vi "Teleop.vi"(10 "Match Info":T1={"Autonomous Elapsed Seconds"=0.0, "TeleOp Elapsed Seconds"=0.0, "Disabled Elapsed Seconds"=0.0, "Visited Autonomous"=FALSE, "Visited TeleOp"=FALSE, "Visited Disabled"=FALSE, "Autonomous Settings"={"Autonomous Style"=enum."Independent", "VI Refnum"=refnum}}, 11 "Call Context":T2) -> ()   [LabVIEW 2015]
doc: "This VI is called for each TeleOp packet received from the DS where the robot is not disabled. It is often used to read from the joysticks and update I/O or to update setpoints for timed control loops. It should complete and return within 20 milliseconds or it may miss DS packets."
uses:
  <vilib>/Rock Robotics/WPI/DriverStation/WPI_DriverStationDerivedRobotMode.ctl
  <vilib>/Rock Robotics/WPI/DriverStation/WPI_DriverStationMatch Info.ctl
  <vilib>/Rock Robotics/WPI/Solenoid/WPI_SolenoidValue.ctl
  <vilib>/Rock Robotics/WPI/CAN/TalonSRX/WPI_CANTalonSRX_BrakeOverride.ctl
  <vilib>/Rock Robotics/WPI/Utilities/WPI_GetSetVariantRefNum.vi
  <vilib>/Rock Robotics/Network Tables/NT Write Boolean Array.vi
  <vilib>/Rock Robotics/Network Tables/NT Write Numeric Array.vi
  <vilib>/Rock Robotics/WPI/Solenoid/WPI_SolenoidSetEnum.vi
  <vilib>/Rock Robotics/Network Tables/NT Read Boolean.vi
  <vilib>/addons/control/pid/pid.llb/PID (DBL).vi
  ADI MXP IMU/ADI MXP IMU/FRC ADI MXP IMU.lvlib
  <vilib>/addons/control/pid/NI_PID_pid.lvlib
panel:
  out "IMU AHRS":cluster{"Pitch":dbl, "Roll":dbl, "Yaw":dbl}
  out "IMU AHRS DELTA":cluster{"Pitch":dbl, "Roll":dbl, "Yaw":dbl}
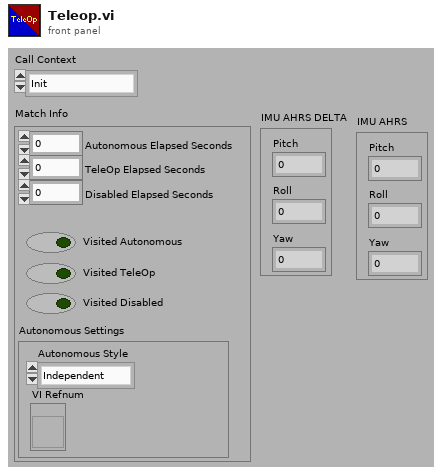
[diagram p1: front panel]
types:
  T1 = typedef "WPI_DriverStationMatch Info.ctl" = cluster{"Autonomous Elapsed Seconds":dbl, "TeleOp Elapsed Seconds":dbl, "Disabled Elapsed Seconds":dbl, "Visited Autonomous":bool, "Visited TeleOp":bool, "Visited Disabled":bool, "Autonomous Settings":cluster{"Autonomous Style":enum16{"Iterative", "Independent"}, "VI Refnum":refnum<vi>}}
  T2 = typedef "WPI_DriverStationDerivedRobotMode.ctl" = enum16{"Init", "Execute", "Stop"}
  T3 = typedef "WPI_CANTalonSRX_BrakeOverride.ctl" = enum8{"No Override", "Override to Coast", "Override to Brake"}
  T4 = typedef "WPI_SolenoidValue.ctl" = enum16{"Off", "On", "Forward", "Reverse"}
  T5 = typedef "WPI_MotorControlDeviceRef.ctl" = cluster{"DeviceStatus":errorcluster, "Type":T6, "PWM":cluster{"PWM Channel":T7, "DeadBand":T8}, "CAN":cluster{"Device Number":u8, "Control Mode":T9, "Semaphore":T10, "Max Vout":dbl, "TalonSRX Control Mode":T11}, "Invert":bool}
  T6 = typedef "WPI_MotorControlType.ctl" = enum16{"PWM", "CAN", "CANTalonSRX"}
  T7 = typedef "FPGA_DIOPWMChannel.ctl" = enum8{"PWM 0", "PWM 1", "PWM 2", "PWM 3", "PWM 4", "PWM 5", "PWM 6", "PWM 7", "PWM 8", "PWM 9", "PWM MXP 0", "PWM MXP 1", "PWM MXP 2", "PWM MXP 3", "PWM MXP 4", "PWM MXP 5", "PWM MXP 6", "PWM MXP 7", "PWM MXP 8", "PWM MXP 9", "Invalid"}
  T8 = typedef "WPI_PWMDeadband.ctl" = cluster{"Name":string, "maxPositivePwm":i32, "minPositivePwm":i32, "centerPwm":i32, "maxNegativePwm":i32, "minNegativePwm":i32, "angularRange":u16}
  T9 = typedef "WPI_CANJaguar_ControlMode.ctl" = enum8{"Percent VBus", "Current", "Speed", "Position", "Voltage"}
  T10 = typedef "Semaphore RefNum" = refnum<k1>
  T11 = typedef "WPI_CANTalonSRX_APIControlMode.ctl" = enum8{"Percent VBus", "Speed", "Position", "Slave", "Unchanged / Invalid", "Voltage Compensation", "Current", "Motion Profile"}
  T12 = typedef "FRC ADI MXP IMU.lvlib/WPI_AnalogDevicesIMUInterruptDevRef.ctl" = cluster{"SimpleGyroDevRef":T13, "InterruptRef":T15}
  T13 = typedef "FRC ADI MXP IMU.lvlib/WPI_AnalogDevicesIMUDevRef.ctl" = cluster{"DevStatus":errorcluster, "Handle":i32, "SPI Bus":T14, "Device Found":bool, "Sample Rate":dbl, "Device Ready":bool, "Yaw Axis":enum16{"X", "Y", "Z"}, "AHRS Algorithm":enum16{"Complementary", "Madgwick"}}
  T14 = typedef "spi_bus.ctl" = enum16{"SPI On-Board, CS0", "SPI On-Board, CS1", "SPI On-Board, CS2", "SPI On-Board, CS3", "SPI MXP", "Invalid"}
  T15 = typedef "WPI_InterruptRef.ctl" = cluster{"DevStatus":errorcluster, "InterruptIndex":T16}
  T16 = typedef "FPGA_InterruptIndex.ctl" = enum8{"0", "1", "2", "3", "4", "5", "6", "7", "Invalid"}
  T17 = typedef "WPI_JoystickDevRef.ctl" = cluster{"Device":T18}
  T18 = typedef "WPI_JoystickDeviceEnum.ctl" = enum16{"USB 0", "USB 1", "USB 2", "USB 3", "USB 4", "USB 5"}
  T19 = cluster{"proportional gain (Kc)":dbl, "integral time (Ti, min)":dbl, "derivative time (Td, min)":dbl}
  T20 = typedef "WPI_SwitchDevRef.ctl" = cluster{"DevStatus":errorcluster, "DIO Channel":T21, "CntIndex":T22, "Normally Closed":bool}
  T21 = typedef "FPGA_DIOChannel.ctl" = enum8{"DIO 0", "DIO 1", "DIO 2", "DIO 3", "DIO 4", "DIO 5", "DIO 6", "DIO 7", "DIO 8", "DIO 9", "DIO MXP 0", "DIO MXP 1", "DIO MXP 2", "DIO MXP 3", "DIO MXP 4", "DIO MXP 5", "DIO MXP 6", "DIO MXP 7", "DIO MXP 8", "DIO MXP 9", "DIO MXP 10", "DIO MXP 11", "DIO MXP 12", "DIO MXP 13", "DIO MXP 14", "DIO MXP 15", "Invalid"}
  T22 = typedef "FPGA_CounterCtrSystemIndex.ctl" = enum8{"Ctr 0", "Ctr 1", "Ctr 2", "Ctr 3", "Ctr 4", "Ctr 5", "Ctr 6", "Ctr 7", "Invalid"}
  T23 = typedef "WPI_SolenoidDevRef.ctl" = cluster{"DevStatus":errorcluster, "Pneumatics Control Module":u8, "Forward Solenoid Channel":T24, "Reverse Solenoid Channel":T24}
  T24 = typedef "WPI_SolenoidChannel.ctl" = enum8{"Solenoid 0", "Solenoid 1", "Solenoid 2", "Solenoid 3", "Solenoid 4", "Solenoid 5", "Solenoid 6", "Solenoid 7", "Invalid"}
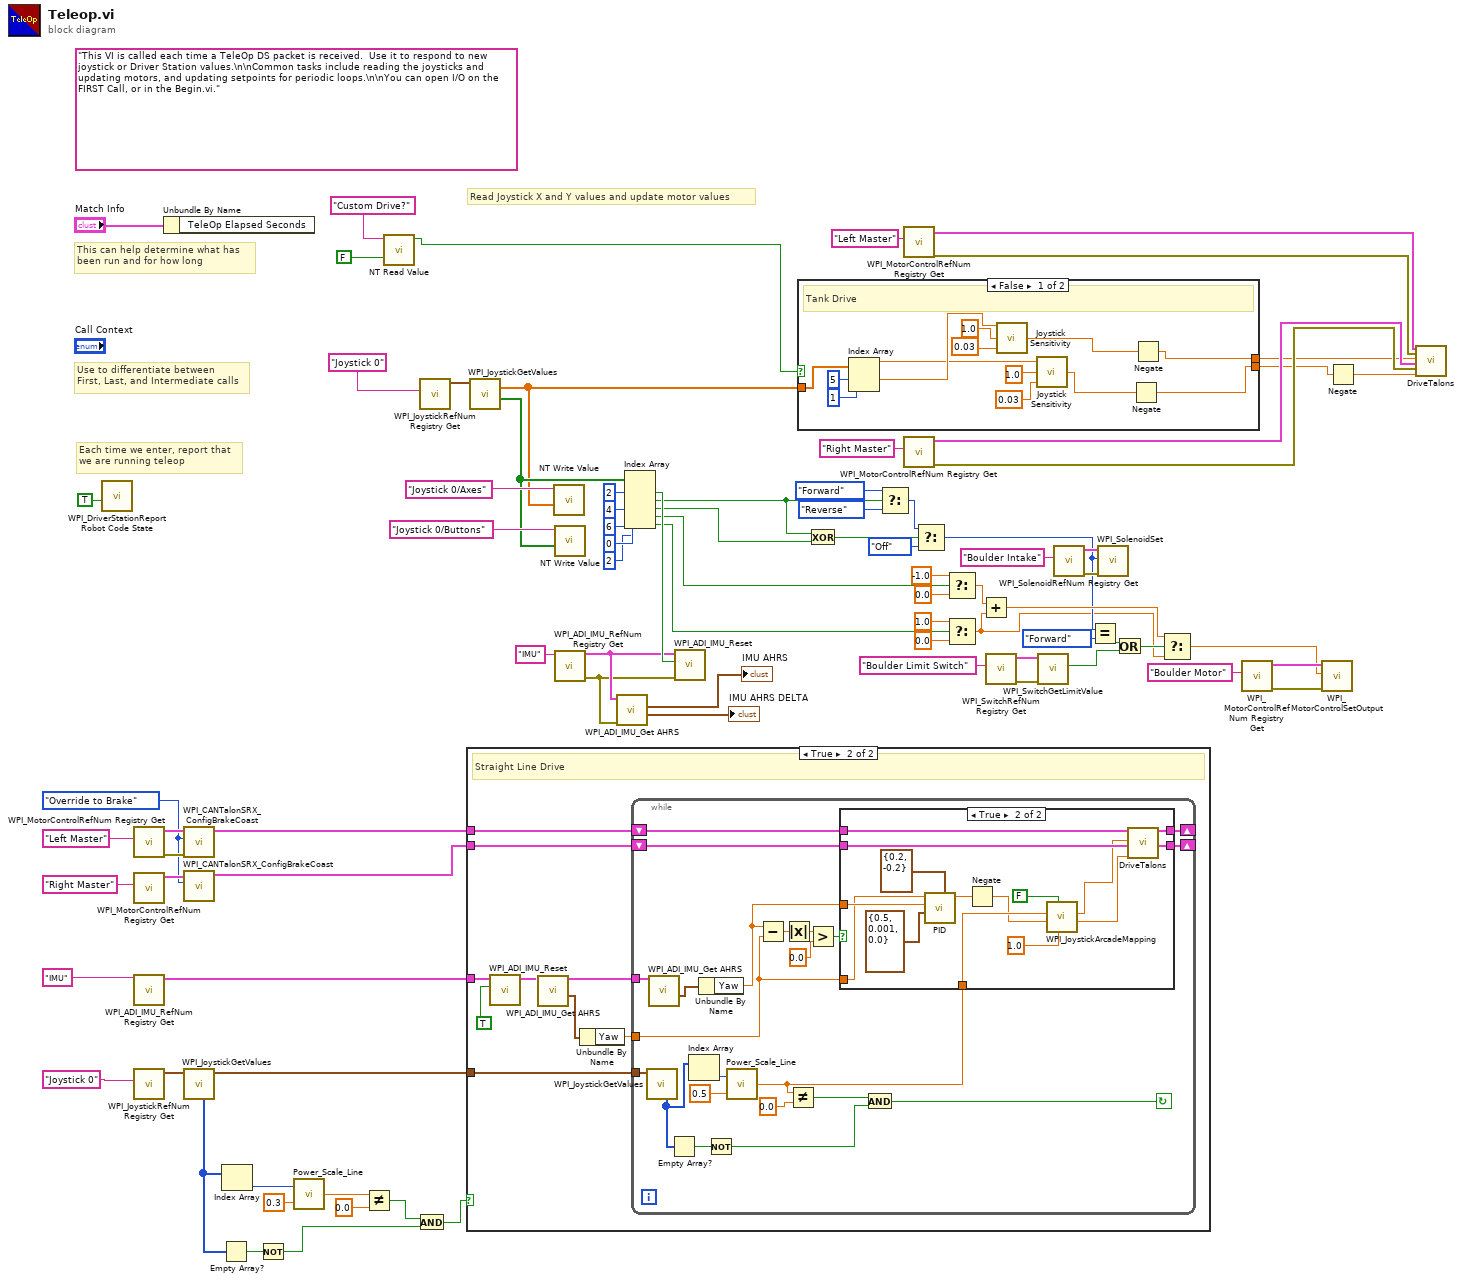
[diagram p0: block diagram]
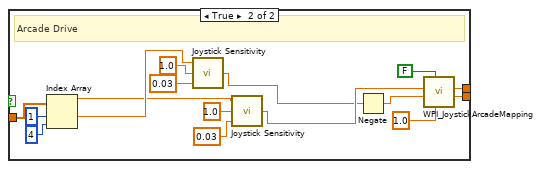
[diagram p2: hidden frame]
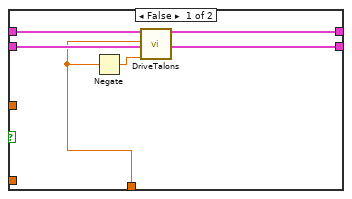
[diagram p4: hidden frame]
diagram:
  w34 = WPI_CANTalonSRX_BrakeOverride."Override to Brake" ("Brake / Coast Mode")
  (unwired) "This VI is called each time a TeleOp DS packet is received.  Use it to respond to new joystick or Driver Station values.\n\nCommon tasks include reading the joysticks and updating motors, and updating setpoints for periodic loops.\n\nYou can open I/O on the FIRST Call, or in the Begin.vi."
  # "Each time we enter, report that\nwe are running teleop"
  # "Use to differentiate between\nFirst, Last, and Intermediate calls"
  # "This can help determine what has\nbeen run and for how long"
  # "Read Joystick X and Y values and update motor values"
  n1 = call <vilib>:"WPI_DriverStationReport Robot Code State.vi"("TeleOp"=TRUE ("Autonomous")) -> ()  [unwired: 10 in, 1 out]
  n2 = call <vilib>:"WPI_MotorControlRefNum Registry Get.vi"("refnum name"="Left Master") -> ("error out"=w36:errorcluster, "MotorControlDevRef"=w37:T5)  [unwired: 9 in]
  n3 = call <vilib>:"WPI_MotorControlRefNum Registry Get.vi"("refnum name"="Right Master") -> ("MotorControlDevRef"=w35:T5)  [unwired: 9 in, 1 out]
  n4 = call "WPI_ADI_IMU_RefNum Registry Get.vi"("refnum name"="IMU") -> ("ADI IMU Interrupt DevRef"=w18:T12)  [unwired: 9 in, 1 out]
  n5 = call <vilib>:"WPI_JoystickRefNum Registry Get.vi"("refnum name"="Joystick 0") -> ("JoystickDevRef"=w13:T17)  [unwired: 1 in, 9 out]
  n6 = Unbundle By Name("Match Info") -> ()  [unwired: 1 out]
  n7 = call <vilib>:"WPI_CANTalonSRX_ConfigBrakeCoast.vi"("error in (no error)"=w36, "Brake / Coast Mode"=w34, "CAN Talon SRX Ref"=w37) -> ("CAN Talon SRX Ref"=w16:T5)  [unwired: 7 in, 1 out]
  n8 = call <vilib>:"WPI_CANTalonSRX_ConfigBrakeCoast.vi"("Brake / Coast Mode"=w34, "CAN Talon SRX Ref"=w35) -> ("CAN Talon SRX Ref"=w17:T5)  [unwired: 8 in, 1 out]
  n9 = call <vilib>:"WPI_JoystickGetValues.vi"("JoystickDevRef"=w13) -> ("JoystickDevRef"=w12:T17, "POVs"=w7:i16[])  [unwired: 6 in, 3 out]
  n10 = Empty Array?(array=w7) -> (empty?=w6:bool)
  n11 = Index Array(array=w7) -> (element=w15:i16)  [unwired: 1 in]
  n12 = Not(x=w6) -> (.not. x?=w5:bool)
  n13 = call "Power_Scale_Line.vi"("Power Input"=0.3, "POV"=w15) -> ("Power Output"=w19:dbl)
  n14 = Not Equal?(x=w19, y=0.0) -> (x != y?=w4:bool)
  n15 = call-poly <vilib>:"NT Read Value.vi"("Default Value"=FALSE, "Name"="Custom Drive?") -> ("Boolean"=w21:bool)  [unwired: 8 in, 1 out]
  n16 = And(x=w4, y=w5) -> (x .and. y?=w3:bool)
  n17 = call <vilib>:"WPI_JoystickRefNum Registry Get.vi"("refnum name"="Joystick 0") -> ("JoystickDevRef"=w31:T17)  [unwired: 1 in, 9 out]
  n18 = case shown="True" w3 {
    tunnel: w18 -> [_ w87]
    tunnel: w17 -> [_ w92]
    tunnel: w16 -> [_ w91]
    tunnel: w12 -> [_ w90]
    frame False {
      # "POV Not Pressed"
    }
    frame True {
      # "Straight Line Drive"
      n19 = call "WPI_ADI_IMU_Reset.vi"("Reset? (T)"=TRUE, "ADI IMU Interrupt DevRef"=w87) -> ("ADI IMU Interrupt DevRef Out"=w86:T12)  [unwired: 8 in, 1 out]
      n20 = call "WPI_ADI_IMU_Get AHRS.vi"("ADI IMU Interrupt DevRef"=w86) -> ("IMU AHRS DELTA"=w88:cluster{"Pitch":dbl, "Roll":dbl, "Yaw":dbl}, "ADI IMU Interrupt DevRef Out"=w89:T12)  [unwired: 6 in, 3 out]
      n21 = Unbundle By Name(w88) -> ("Yaw"=w93:dbl)
      n22 = while {
        tunnel: w89 -> [w97]
        tunnel: w93 -> [w106]
        shift-right: [w111] -> _
        shift-left: w92 -> [w110]
        shift-right: [w112] -> _
        shift-left: w91 -> [w109]
        tunnel: w90 -> [w103]
        stop <- w99 continue-if-true
        n23 = call <vilib>:"WPI_JoystickGetValues.vi"("JoystickDevRef"=w103) -> ("POVs"=w98:i16[])  [unwired: 6 in, 4 out]
        n24 = call "WPI_ADI_IMU_Get AHRS.vi"("ADI IMU Interrupt DevRef"=w97) -> ("IMU AHRS DELTA"=w96:cluster{"Pitch":dbl, "Roll":dbl, "Yaw":dbl})  [unwired: 6 in, 4 out]
        n25 = Empty Array?(array=w98) -> (empty?=w102:bool)
        n26 = Index Array(array=w98) -> (element=w113:i16)  [unwired: 1 in]
        n27 = Unbundle By Name(w96) -> ("Yaw"=w107:dbl)
        n28 = Not(x=w102) -> (.not. x?=w101:bool)
        n29 = call "Power_Scale_Line.vi"("Power Input"=0.5, "POV"=w113) -> ("Power Output"=w108:dbl)
        n30 = Subtract(x=w107, y=w106) -> (x-y=w95:dbl)
        n31 = Absolute Value(x=w95) -> (abs(x)=w94:dbl)
        n32 = Not Equal?(x=w108, y=0.0) -> (x != y?=w100:bool)
        n33 = Greater?(x=w94, y=0.0) -> (0:w104:bool)
        n34 = case shown="True" w104 {
          tunnel: [w121 w136] -> w112
          tunnel: [w120 w135] -> w111
          tunnel: w110 -> [w118 w134]
          tunnel: w109 -> [w119 w133]
          tunnel: w108 -> [w116 w125]
          tunnel: w107 -> [_ w132]
          tunnel: w106 -> [_ w131]
          frame False {
            n35 = Negate(x=w116) -> (-x=w117:dbl)
            n36 = call "DriveTalons.vi"("Left Motor"=w119, "Left Stick"=w116, "Right Motor"=w118, "Right Stick"=w117) -> ("Left Motor Out"=w121:T5, "Right Motor Out"=w120:T5)  [unwired: 12 in, 2 out]
          }
          frame True {
            n37 = call-poly <vilib>:"PID.vi"("output range"=cluster{"output high":dbl, "output low":dbl} {"output high"=0.2, "output low"=-0.2}, "PID gains"=T19 {"proportional gain (Kc)"=0.5, "integral time (Ti, min)"=0.001, "derivative time (Td, min)"=0.0}, "process variable"=w132, "setpoint"=w131) -> ("output"=w124:dbl)  [unwired: 6 in, 1 out]
            n38 = Negate(x=w124) -> (-x=w123:dbl)
            n39 = call <vilib>:"WPI_JoystickArcadeMapping.vi"("Max Output"=1.0, "Square Inputs"=FALSE, "Y axis value"=w123, "X axis value"=w125) -> ("Right Motor Value"=w126:dbl, "Left Motor Value"=w122:dbl)  [unwired: 6 in]
            n40 = call "DriveTalons.vi"("Left Motor"=w133, "Left Stick"=w122, "Right Motor"=w134, "Right Stick"=w126) -> ("Left Motor Out"=w136:T5, "Right Motor Out"=w135:T5)  [unwired: 12 in, 2 out]
          }
        }
        n41 = And(x=w100, y=w101) -> (x .and. y?=w99:bool)
      }
    }
  }
  n42 = call <vilib>:"WPI_JoystickGetValues.vi"("JoystickDevRef"=w31) -> ("Buttons"=w78:bool[], "Axes"=w20:dbl[])  [unwired: 6 in, 3 out]
  n43 = call-poly <vilib>:"NT Write Value.vi"("Numeric Array"=w20, "Name"="Joystick 0/Axes") -> ()  [unwired: 9 in, 1 out]
  n44 = call-poly <vilib>:"NT Write Value.vi"("Boolean Array"=w78, "Name"="Joystick 0/Buttons") -> ()  [unwired: 9 in, 1 out]
  n45 = call "WPI_ADI_IMU_RefNum Registry Get.vi"("refnum name"="IMU") -> ("error out"=w10:errorcluster, "ADI IMU Interrupt DevRef"=w11:T12)  [unwired: 9 in]
  n46 = call "WPI_ADI_IMU_Get AHRS.vi"("error in"=w10, "ADI IMU Interrupt DevRef"=w11) -> ("IMU AHRS DELTA"=→"IMU AHRS DELTA":cluster{"Pitch":dbl, "Roll":dbl, "Yaw":dbl}, "IMU AHRS"=→"IMU AHRS":cluster{"Pitch":dbl, "Roll":dbl, "Yaw":dbl})  [unwired: 5 in, 3 out]
  n47 = Index Array(array=w78, index #1=2 ("index"), index #2=4 ("index"), index #3=6 ("index"), index #4=0 ("index"), index #5=2 ("index")) -> (element #1=w76:bool, element #2=w41:bool, element #3=w42:bool, element #4=w53:bool, element #5=w52:bool)
  n48 = call "WPI_ADI_IMU_Reset.vi"("error in"=w10, "Reset? (T)"=w76, "ADI IMU Interrupt DevRef"=w11) -> ()  [unwired: 7 in, 2 out]
  n49 = case shown="False" w21 {
    tunnel: [w139 w163] -> w22
    tunnel: [w137 w162] -> w2
    tunnel: w20 -> [w147 w159]
    frame False {
      # "Tank Drive"
      n50 = Index Array(array=w147, index #1=5 ("index"), index #2=1 ("index")) -> (element #1=w146:dbl, element #2=w143:dbl)
      n51 = call "Joystick Sensitivity.vi"("B"=0.03, "A"=1.0, "X"=w146) -> ("Y"=w140:dbl)
      n52 = call "Joystick Sensitivity.vi"("B"=0.03, "A"=1.0, "X"=w143) -> ("Y"=w138:dbl)
      n53 = Negate(x=w138) -> (-x=w137:dbl)
      n54 = Negate(x=w140) -> (-x=w139:dbl)
    }
    frame True {
      # "Arcade Drive"
      n55 = Index Array(array=w159, index #1=1 ("index"), index #2=4 ("index")) -> (element #1=w158:dbl, element #2=w155:dbl)
      n56 = call "Joystick Sensitivity.vi"("B"=0.03, "A"=1.0, "X"=w158) -> ("Y"=w151:dbl)
      n57 = call "Joystick Sensitivity.vi"("B"=0.03, "A"=1.0, "X"=w155) -> ("Y"=w152:dbl)
      n58 = Negate(x=w151) -> (-x=w150:dbl)
      n59 = call <vilib>:"WPI_JoystickArcadeMapping.vi"("Max Output"=1.0, "Square Inputs"=FALSE, "Y axis value"=w150, "X axis value"=w152) -> ("Right Motor Value"=w162:dbl, "Left Motor Value"=w163:dbl)  [unwired: 6 in]
    }
  }
  n60 = Exclusive Or(1:w42, 2:w41) -> (0:w49:bool)
  n61 = Select(t=WPI_SolenoidValue."Forward", s=w41, f=WPI_SolenoidValue."Reverse" ("Value")) -> (s? t:f=w48:T4)
  n62 = call <vilib>:"WPI_MotorControlRefNum Registry Get.vi"("refnum name"="Left Master") -> ("error out"=w25:errorcluster, "MotorControlDevRef"=w26:T5)  [unwired: 9 in]
  n63 = call <vilib>:"WPI_MotorControlRefNum Registry Get.vi"("refnum name"="Right Master") -> ("error out"=w23:errorcluster, "MotorControlDevRef"=w24:T5)  [unwired: 9 in]
  n64 = Select(t=w48, s=w49, f=WPI_SolenoidValue."Off") -> (s? t:f=w45:T4)
  n65 = Select(t=-1.0, s=w53, f=0.0) -> (s? t:f=w64:dbl)
  n66 = Select(t=1.0, s=w52, f=0.0) -> (s? t:f=w43:dbl)
  n67 = Add(x=w64, y=w43) -> (x+y=w46:dbl)
  n68 = call <vilib>:"WPI_SwitchRefNum Registry Get.vi"("refnum name"="Boulder Limit Switch") -> ("error out"=w57:errorcluster, "SwitchDevRef"=w56:T20)  [unwired: 9 in]
  n69 = call <vilib>:"WPI_SwitchGetLimitValue.vi"("error in (no error)"=w57, "SwitchDevRef"=w56) -> ("Switch Pressed"=w44:bool)  [unwired: 7 in, 2 out]
  n70 = call <vilib>:"WPI_SolenoidRefNum Registry Get.vi"("refnum name"="Boulder Intake") -> ("error out"=w63:errorcluster, "SolenoidDevRef"=w62:T23)  [unwired: 9 in]
  n71 = Equal?(x=w45, y=WPI_SolenoidValue."Forward" ("Value")) -> (x = y?=w55:bool)
  n72 = call-poly <vilib>:"WPI_SolenoidSet.vi"("error in (no error)"=w63, "Value"=w45, "SolenoidDevRef"=w62) -> ()  [unwired: 7 in, 2 out]
  n73 = Or(x=w55, y=w44) -> (x .or. y?=w59:bool)
  n74 = Select(t=w46, s=w59, f=w43) -> (s? t:f=w60:dbl)
  n75 = call <vilib>:"WPI_MotorControlRefNum Registry Get.vi"("refnum name"="Boulder Motor") -> ("error out"=w69:errorcluster, "MotorControlDevRef"=w70:T5)  [unwired: 9 in]
  n76 = call <vilib>:"WPI_MotorControlSetOutput.vi"("error in (no error)"=w69, "Output"=w60, "MotorControlDevRef"=w70) -> ()  [unwired: 6 in, 3 out]
  n77 = Negate(x=w2) -> (-x=w1:dbl)
  n78 = call "DriveTalons.vi"("Left Motor"=w26, "Left Motor Error"=w25, "Left Stick"=w22, "Right Motor"=w24, "Right Motor Error"=w23, "Right Stick"=w1) -> ()  [unwired: 10 in, 4 out]
